vi "SEA-9510 RT.vi"() -> ()   [LabVIEW 2019]
panel:
  out "Ch1 Position":u64
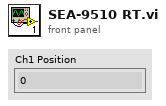
[diagram p1: front panel]
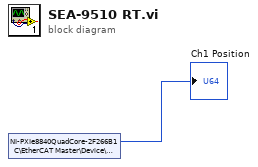
[diagram p0: block diagram]
diagram:
  n1 = shared-variable "NI-PXIe8840QuadCore-2F266B1C\\EtherCAT Master\\Device\\User-Defined Variables\\Ch1 Position"() -> (→"Ch1 Position":u64)  [unwired: 1 in, 1 out]
